vi "Make VI Param(Read Batch Profile Rsp).vi"(1 "pRsp":T1) -> (0 "Read Batch Profile Rsp":T2)   [LabVIEW 2014, in "Keyence LJ-V7000.lvlib"]
uses:
  Keyence LJ-V7000.lvlib
  Public/Clusters/Read Batch Profile Rsp.ctl
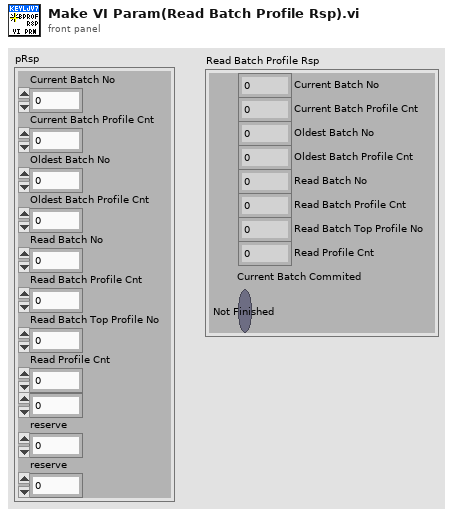
[diagram p1: front panel]
types:
  T1 = cluster{"Current Batch No":u32, "Current Batch Profile Cnt":u32, "Oldest Batch No":u32, "Oldest Batch Profile Cnt":u32, "Read Batch No":u32, "Read Batch Profile Cnt":u32, "Read Batch Top Profile No":u32, "Read Profile Cnt":u8, u8, "reserve":u8, "reserve":u8}
  T2 = typedef "Keyence LJ-V7000.lvlib/Read Batch Profile Rsp.ctl" = cluster{"Current Batch No":u32, "Current Batch Profile Cnt":u32, "Oldest Batch No":u32, "Oldest Batch Profile Cnt":u32, "Read Batch No":u32, "Read Batch Profile Cnt":u32, "Read Batch Top Profile No":u32, "Read Profile Cnt":u8, "Current Batch Commited":bool}
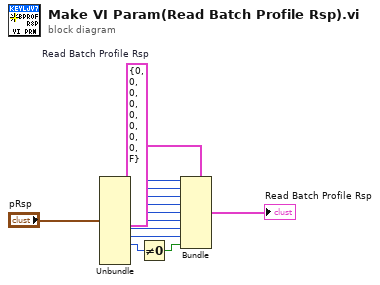
[diagram p0: block diagram]
diagram:
  w9 = T2 {"Current Batch No"=0, "Current Batch Profile Cnt"=0, "Oldest Batch No"=0, "Oldest Batch Profile Cnt"=0, "Read Batch No"=0, "Read Batch Profile Cnt"=0, "Read Batch Top Profile No"=0, "Read Profile Cnt"=0, "Current Batch Commited"=FALSE}  # Read Batch Profile Rsp
  n1 = Unbundle("pRsp") -> ("Current Batch No"=w13:u32, "Current Batch Profile Cnt"=w12:u32, "Oldest Batch No"=w11:u32, "Oldest Batch Profile Cnt"=w10:u32, "Read Batch No"=w8:u32, "Read Batch Profile Cnt"=w7:u32, "Read Batch Top Profile No"=w6:u32, "Read Profile Cnt"=w5:u8, w4:u8)  [unwired: 2 out]
  n2 = Not Equal To 0?(x=w4) -> (x != 0?=w3:bool)
  n3 = Bundle(cluster=w9, "Current Batch No"=w13, "Current Batch Profile Cnt"=w12, "Oldest Batch No"=w11, "Oldest Batch Profile Cnt"=w10, "Read Batch No"=w8, "Read Batch Profile Cnt"=w7, "Read Batch Top Profile No"=w6, "Read Profile Cnt"=w5, "Current Batch Commited"=w3) -> (→"Read Batch Profile Rsp":T2)
